vi "TableAutosizeColumnsFromHeaders.vi"(11 "Table in":refnum<vi>) -> ()   [LabVIEW 2026]
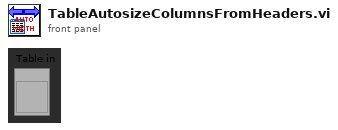
[diagram p1: front panel]
types:
  T1 = cluster{"Font Name:":string, "Size":i16, "Strikeout?":bool, "Italic?":bool, "Underline?":bool, "Outline?":bool, "Shadow?":bool, "Bold?":bool}
  T2 = enum16{"User-specified Font", "Application Font", "System Font", "Dialog Font"}
  T3 = typedef "LVFontTypeDef.ctl" = cluster{"Font Name":string, "Size":u16, "Bold":bool, "Italic":bool, "Underline":bool, "Strikeout":bool, "Color":u32}
  T4 = cluster{"left":i16, "top":i16, "right":i16, "bottom":i16}
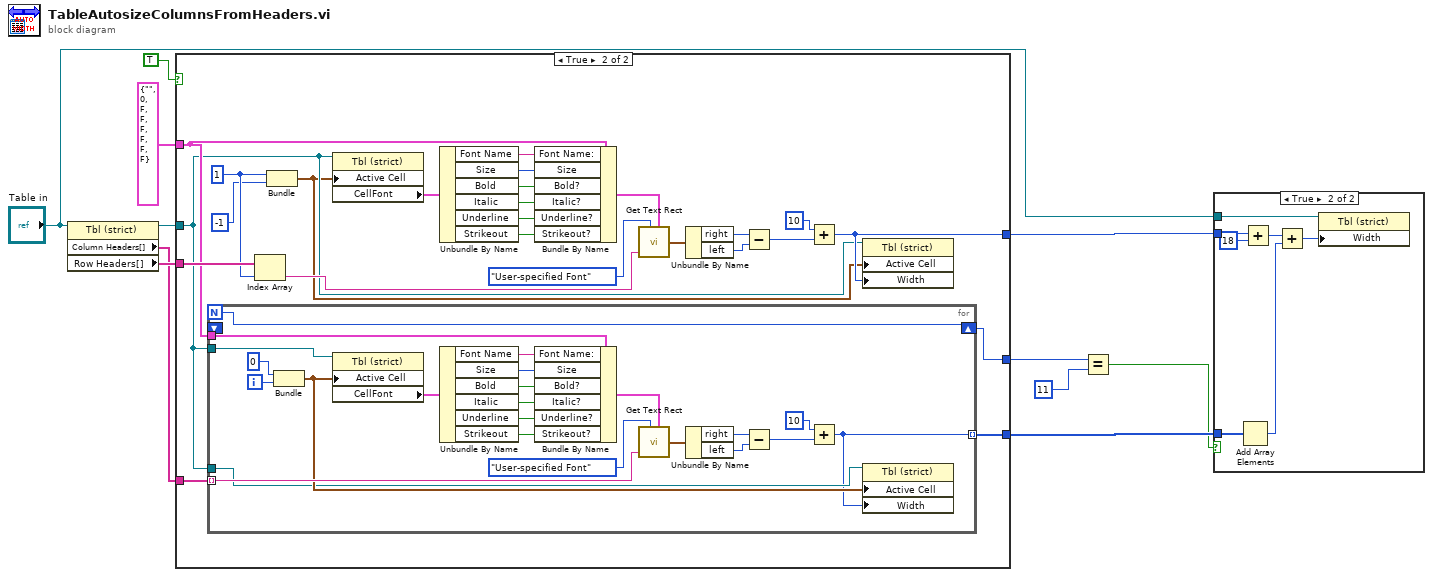
[diagram p0: block diagram]
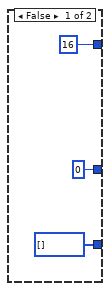
[diagram p3: hidden frame]
diagram:
  n1 = property class="Tbl (strict)"(reference="Table in") -> (reference out=w8:refnum<vi>, "Column Headers[]"=w7:string[], "Row Headers[]"=w9:string[])  [unwired: 1 in, 1 out]
  n2 = case shown="True" TRUE {
    tunnel: w8 -> [_ w18]
    tunnel: T1 {"Font Name:"="", "Size"=0, "Strikeout?"=FALSE, "Italic?"=FALSE, "Underline?"=FALSE, "Outline?"=FALSE, "Shadow?"=FALSE, "Bold?"=FALSE} ("[user-specified font]") -> [_ w21]
    tunnel: w9 -> [_ w31]
    tunnel: [16 w19] -> w6
    tunnel: w7 -> [_ w20]
    tunnel: [i16[] [] w17] -> w4
    tunnel: [0 w16] -> w3
    frame False {
    }
    frame True {
      w30 = 1
      n3 = for {
        N -> [w40]
        tunnel: w21 -> [w53]
        tunnel: w20 -> [w51] mode=indexing
        tunnel: w18 -> [w46]
        tunnel: w18 -> [w44]
        tunnel: [w41] -> w17 mode=indexing
        shift-right: [w40] -> w16
        shift-left: _ -> [_]
        i -> [w62]
        n4 = Bundle(0, w62) -> (w45:cluster{i32, i32})  [unwired: 1 in]
        n5 = property class="Tbl (strict)"(reference=w46, "Active Cell"=w45) -> ("CellFont"=w60:T3)  [unwired: 1 in, 2 out]
        n6 = Unbundle By Name(w60) -> ("Font Name"=w59:string, "Size"=w58:u16, "Bold"=w57:bool, "Italic"=w56:bool, "Underline"=w55:bool, "Strikeout"=w54:bool)
        n7 = Bundle By Name(cluster=w53, "Font Name:"=w59, "Size"=w58, "Bold?"=w57, "Italic?"=w56, "Underline?"=w55, "Strikeout?"=w54) -> (w52:T1)
        n8 = call <vilib>:"Get Text Rect.vi"("desired font(Application)"=T2."User-specified Font", "text"=w51, "[user-specified font]"=w52) -> ("rect"=w49:T4)  [unwired: 6 in]
        n9 = Unbundle By Name(w49) -> ("right"=w48:i16, "left"=w47:i16)
        n10 = Subtract(x=w48, y=w47) -> (x-y=w43:i16)
        n11 = Add(x=i16 10, y=w43) -> (x+y=w41:i16)
        n12 = property class="Tbl (strict)"(reference=w44, "Active Cell"=w45, "Width"=w41) -> ()  [unwired: 1 in, 2 out]
      }
      n13 = Index Array(array=w31, index=w30) -> (element=w28:string)
      n14 = Bundle(w30, -1) -> (w15:cluster{i32, i32})  [unwired: 1 in]
      n15 = property class="Tbl (strict)"(reference=w18, "Active Cell"=w15) -> ("CellFont"=w22:T3)  [unwired: 1 in, 2 out]
      n16 = Unbundle By Name(w22) -> ("Font Name"=w39:string, "Size"=w38:u16, "Bold"=w37:bool, "Italic"=w36:bool, "Underline"=w35:bool, "Strikeout"=w34:bool)
      n17 = Bundle By Name(cluster=w21, "Font Name:"=w39, "Size"=w38, "Bold?"=w37, "Italic?"=w36, "Underline?"=w35, "Strikeout?"=w34) -> (w32:T1)
      n18 = call <vilib>:"Get Text Rect.vi"("desired font(Application)"=T2."User-specified Font", "text"=w28, "[user-specified font]"=w32) -> ("rect"=w23:T4)  [unwired: 6 in]
      n19 = Unbundle By Name(w23) -> ("right"=w27:i16, "left"=w26:i16)
      n20 = Subtract(x=w27, y=w26) -> (x-y=w25:i16)
      n21 = Add(x=i16 10, y=w25) -> (x+y=w19:i16)
      n22 = property class="Tbl (strict)"(reference=w18, "Active Cell"=w15, "Width"=w19) -> ()  [unwired: 1 in, 2 out]
    }
  }
  n23 = Equal?(x=w3, y=11) -> (x = y?=w1:bool)
  n24 = case shown="True" w1 {
    tunnel: w6 -> [_ w64]
    tunnel: "Table in" -> [_ w67]
    tunnel: w4 -> [_ w66]
    frame False {
    }
    frame True {
      n25 = Add Array Elements(numeric array=w66) -> (sum=w69:i16)
      n26 = Add(x=w64, y=18) -> (x+y=w65:i32)
      n27 = Add(x=w65, y=w69) -> (x+y=w68:i32)
      n28 = property class="Tbl (strict)"(reference=w67, "Width"=w68) -> ()  [unwired: 1 in, 2 out]
    }
  }
